vi "Run_Core.vi"(0 "Message Popup in":refnum<class "Numeric Functions.lvclass">, 11 "error in (no error)":errorcluster) -> (4 "Message Popup out":refnum<class "Numeric Functions.lvclass">, 6 "Return":variant, 15 "error out":errorcluster)   [LabVIEW 2016, in "Numeric Functions.lvclass"]
uses:
  Numeric Functions.lvclass
  Numeric Functions.lvclass/Numeric Functions.ctl
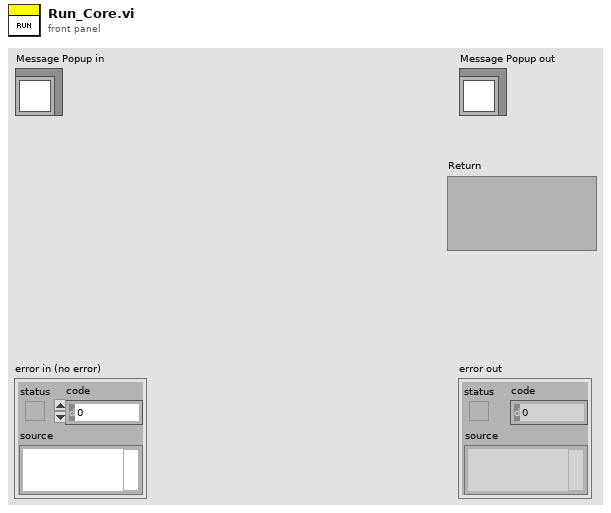
[diagram p1: front panel]
types:
  T1 = typedef "Numeric Functions.lvclass/Function List.ctl" = enum16{"Add", "Sub", "Multiply", "Divide", "Modulus", "Increament", "Decrement", "Square Root", "Square", "Negate", "Reciprocal", "Random Number"}
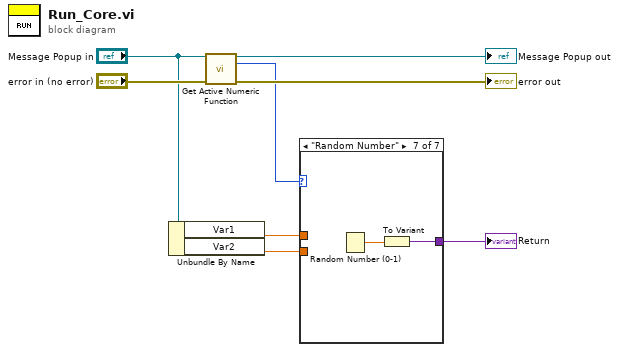
[diagram p0: block diagram]
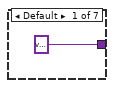
[diagram p2: hidden frame]
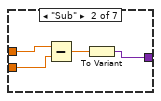
[diagram p3: hidden frame]
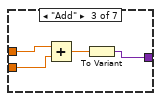
[diagram p4: hidden frame]
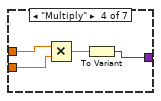
[diagram p5: hidden frame]
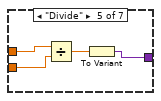
[diagram p6: hidden frame]
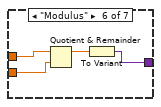
[diagram p7: hidden frame]
diagram:
  n1 = Unbundle By Name("Message Popup in") -> ("Var1"=w8:dbl, "Var2"=w7:dbl)
  n2 = call "Get Active Numeric Function.vi"("Numeric Functions in"="Message Popup in", "error in (no error)"="error in (no error)") -> ("Numeric Functions out"=→"Message Popup out":refnum<class "Numeric Functions.lvclass">, "Function"=w1:T1, "error out"=→"error out":errorcluster)  [unwired: 11 in]
  n3 = case shown="\"Random Number\"" w1 {
    tunnel: w8 -> [_ w13 w17 w21 w25 w29 _]
    tunnel: w7 -> [_ w12 w16 w20 w24 w28 _]
    tunnel: [variant ("Variant") w10 w14 w18 w22 w27 w30] -> w6
    frame Default {
    }
    frame "Sub" {
      n4 = Subtract(x=w13, y=w12) -> (x-y=w11:dbl)
      n5 = To Variant(anything=w11) -> (Variant=w10:variant)
    }
    frame "Add" {
      n6 = Add(x=w17, y=w16) -> (x+y=w15:dbl)
      n7 = To Variant(anything=w15) -> (Variant=w14:variant)
    }
    frame "Multiply" {
      n8 = Multiply(x=w21, y=w20) -> (x*y=w19:dbl)
      n9 = To Variant(anything=w19) -> (Variant=w18:variant)
    }
    frame "Divide" {
      n10 = Divide(x=w25, y=w24) -> (x/y=w23:dbl)
      n11 = To Variant(anything=w23) -> (Variant=w22:variant)
    }
    frame "Modulus" {
      n12 = Quotient & Remainder(x=w29, y=w28) -> (x-y*floor(x/y)=w26:dbl)  [unwired: 1 out]
      n13 = To Variant(anything=w26) -> (Variant=w27:variant)
    }
    frame "Random Number" {
      n14 = Random Number (0-1)() -> (number: 0 to 1=w31:dbl)
      n15 = To Variant(anything=w31) -> (Variant=w30:variant)
    }
  }
  "Return" <- w6
